vi "FFT and LP.vi"(8 "Threshold":dbl, 11 "Data In":dbl[][](array[numeric])) -> (3 "Data Out":dbl[][](array[numeric]))   [LabVIEW 2015]
uses:
  <vilib>/Analysis/2dsp.llb/2D Real FFT.vi
  <vilib>/Analysis/2dsp.llb/2D Inverse Complex FFT.vi
  <vilib>/Analysis/NI_AALPro.lvlib
panel:
  out "Intensity Graph 3":dbl[][](graph)
  out "size(s)":i32
  out "FFT {X}":cdb[][](array[numeric])
  out "Intensity Graph 2":dbl[][](graph)
  out "Intensity Graph":dbl[][](graph)
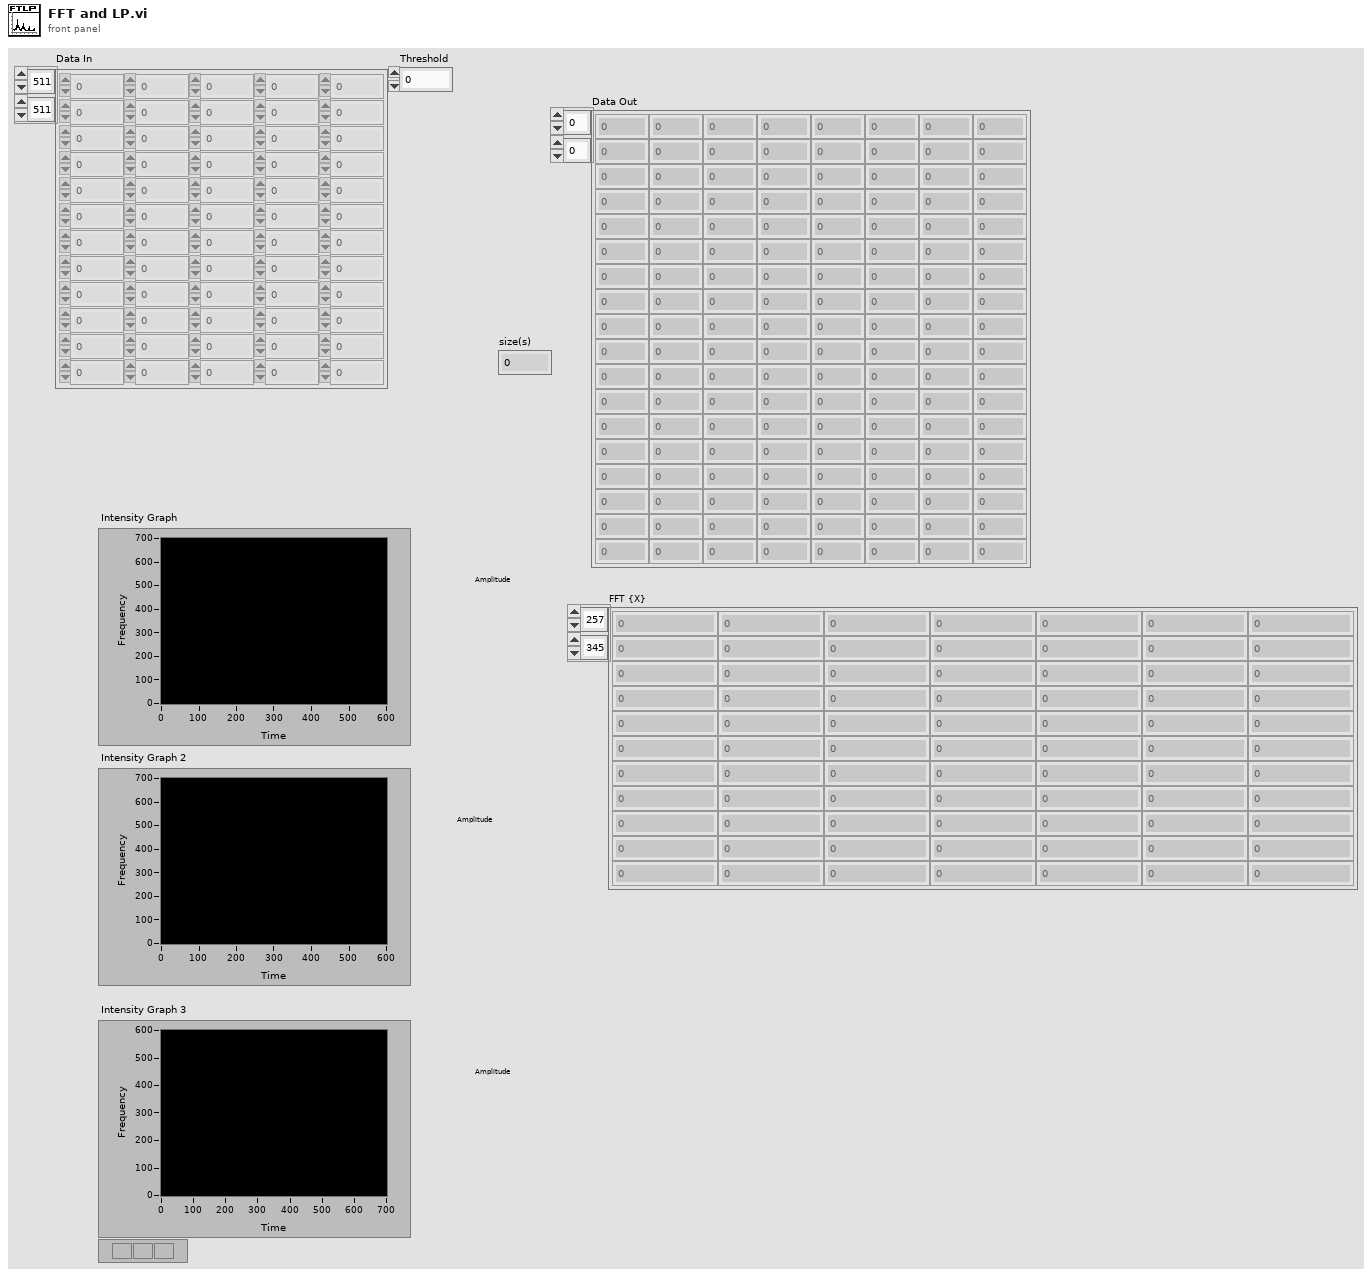
[diagram p1: front panel]
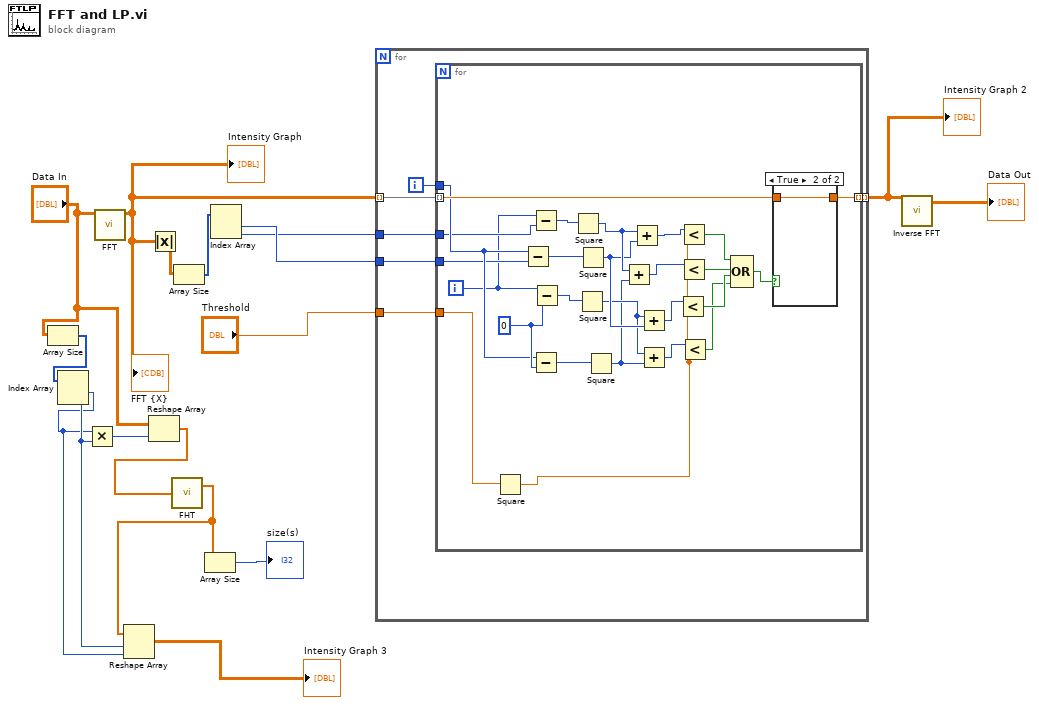
[diagram p0: block diagram]
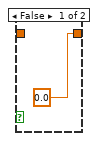
[diagram p2: hidden frame]
diagram:
  n1 = Array Size(array="Data In") -> (size(s)=w9:i32[])
  n2 = Index Array(array=w9) -> (element #1=w1:i32, element #2=w2:i32)  [unwired: 2 in]
  n3 = Multiply(x=w1, y=w2) -> (x*y=w7:i32)
  n4 = call-poly <vilib>:"FFT.vi"("X"="Data In") -> ("FFT {X}"=w11:cdb[][])  [unwired: 9 in, 1 out]
  "Intensity Graph" <- w11
  "FFT {X}" <- w11
  n5 = Reshape Array("Data In", w7) -> (w6:dbl[])
  n6 = Absolute Value(x=w11) -> (abs(x)=w14:dbl[][])
  n7 = call <vilib>:"FHT.vi"("X"=w6) -> ("Hartley {X}"=w4:dbl[])  [unwired: 1 out]
  n8 = Reshape Array(w4, w2, w1) -> (→"Intensity Graph 3":dbl[][])
  n9 = Array Size(array=w14) -> (size(s)=w17:i32[])
  n10 = Array Size(array=w4) -> (size(s)=→"size(s)":i32)
  n11 = Index Array(array=w17) -> (element #1=w13:i32, element #2=w12:i32)  [unwired: 2 in]
  n12 = for {
    tunnel: w11 -> [w23] mode=indexing
    tunnel: "Threshold" -> [w21]
    tunnel: [w20] -> w10 mode=indexing
    tunnel: w13 -> [w19]
    tunnel: w12 -> [w18]
    i -> [w22]
    n13 = for {
      tunnel: w23 -> [w46] mode=indexing
      tunnel: w22 -> [w42]
      tunnel: w21 -> [w49]
      tunnel: [w45] -> w20 mode=indexing
      tunnel: w19 -> [w41]
      tunnel: w18 -> [w39]
      i -> [w38]
      w43 = 0 ("y")
      n14 = Square(x=w49) -> (x^2=w33:dbl)
      n15 = Subtract(x=w42, y=w41) -> (x-y=w48:i32)
      n16 = Subtract(x=w38, y=w39) -> (x-y=w40:i32)
      n17 = Subtract(x=w42, y=w43) -> (x-y=w44:i32)
      n18 = Subtract(x=w38, y=w43) -> (x-y=w47:i32)
      n19 = Square(x=w40) -> (x^2=w37:i32)
      n20 = Square(x=w47) -> (x^2=w35:i32)
      n21 = Square(x=w48) -> (x^2=w36:i32)
      n22 = Square(x=w44) -> (x^2=w34:i32)
      n23 = Add(x=w37, y=w34) -> (x+y=w31:i32)
      n24 = Add(x=w37, y=w36) -> (x+y=w32:i32)
      n25 = Add(x=w35, y=w36) -> (x+y=w30:i32)
      n26 = Add(x=w35, y=w34) -> (x+y=w29:i32)
      n27 = Less?(x=w30, y=w33) -> (x < y?=w26:bool)
      n28 = Less?(x=w32, y=w33) -> (x < y?=w28:bool)
      n29 = Less?(x=w31, y=w33) -> (x < y?=w27:bool)
      n30 = Less?(x=w29, y=w33) -> (x < y?=w25:bool)
      n31 = Compound Arithmetic op=OR(w28, w27, w26, w25) -> (w24:bool)
      n32 = case shown="True" w24 {
        tunnel: w46 -> [_ w51]
        tunnel: [0.0 w51] -> w45
        frame False {
        }
        frame True {
        }
      }
    }
  }
  "Intensity Graph 2" <- w10
  n33 = call-poly <vilib>:"Inverse FFT.vi"("FFT {x}"=w10) -> ("X"=→"Data Out":cdb[][])  [unwired: 9 in, 1 out]
